vi "FPGA2_EPTDigChannels_eDIDS.vi"(0 "NI 9411-3/DI5:0":u8, 1 "VRHall-1.Data":T3 caption="VRHall_Data", 2 "9411-3.Invert":u8, 3 "VRHall-1.Invert":u8, 4 "9411-3.FilterValues":T2, 5 "VRHall-1.FilterValues":T4) -> (8 "9411-3.0.PPWData":T1, 9 "VRHall-1.1.PPWData":T1, 10 "9411-3.1.PPWData":T1, 11 "VRHall-1.2.PPWData":T1, 12 "9411-3.2.PPWData":T1, 13 "VRHall-1.3.PPWData":T1, 14 "9411-3.3.PPWData":T1, 15 "VRHall-1.4.PPWData":T1, 16 "9411-3.4.PPWData":T1, 17 "VRHall-1.5.PPWData":T1, 18 "9411-3.5.PPWData":T1, 19 "VRHall-1.6.PPWData":T1, 20 "9411-3.DigitalTriggers":bool[](array[boolean]), 21 "VRHall-1.DigitalTriggers":bool[](array[boolean]))   [LabVIEW 2015, in "ECS-FPGA.lvlib"]
uses:
  ECS-FPGA.lvlib
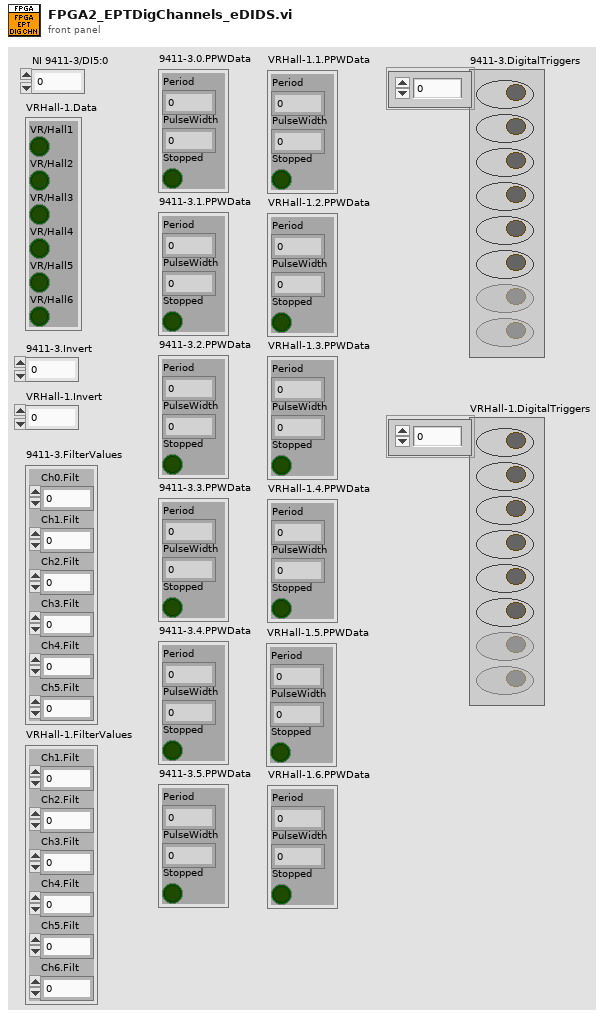
[diagram p1: front panel]
types:
  T1 = cluster{"Period":u32, "PulseWidth":u32, "Stopped":bool}
  T2 = cluster{"Ch0.Filt":u16, "Ch1.Filt":u16, "Ch2.Filt":u16, "Ch3.Filt":u16, "Ch4.Filt":u16, "Ch5.Filt":u16}
  T3 = cluster{"VR/Hall1":bool, "VR/Hall2":bool, "VR/Hall3":bool, "VR/Hall4":bool, "VR/Hall5":bool, "VR/Hall6":bool}
  T4 = cluster{"Ch1.Filt":u16, "Ch2.Filt":u16, "Ch3.Filt":u16, "Ch4.Filt":u16, "Ch5.Filt":u16, "Ch6.Filt":u16}
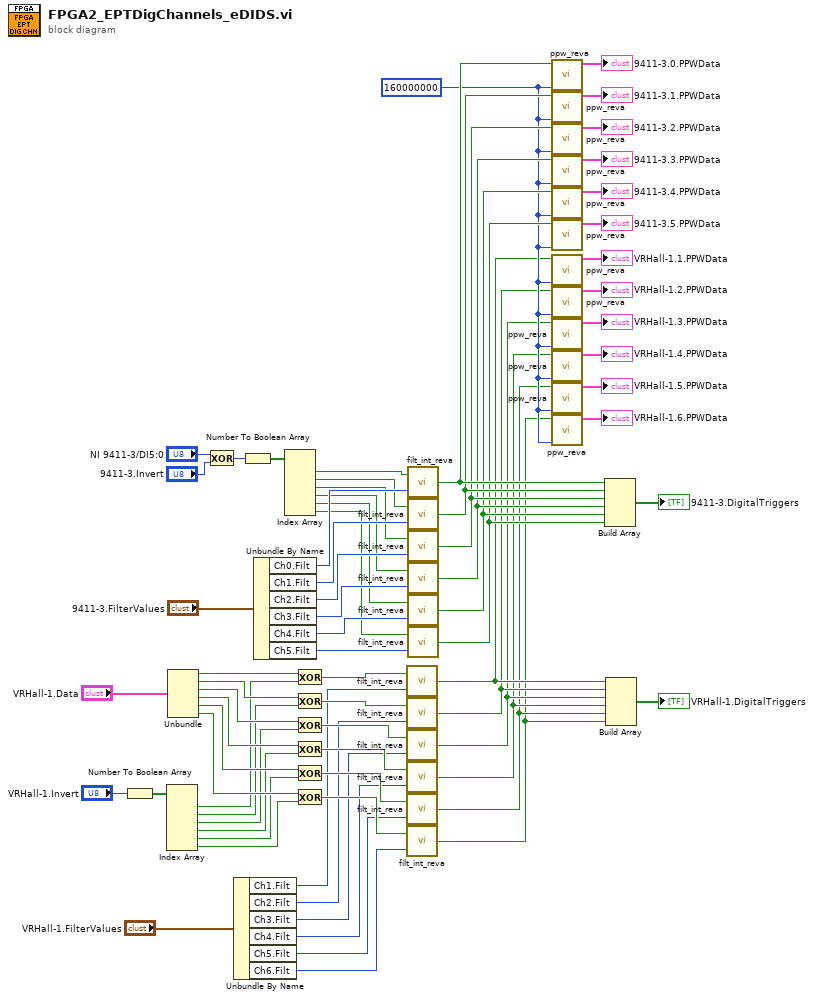
[diagram p0: block diagram]
diagram:
  w32 = u32 160000000 ("StopValue")
  n1 = Number To Boolean Array(number="VRHall-1.Invert") -> (Boolean array=w58:bool[])
  n2 = Index Array(array=w58) -> (element #1=w51:bool, element #2=w50:bool, element #3=w49:bool, element #4=w48:bool, element #5=w47:bool, element #6=w46:bool)  [unwired: 6 in]
  n3 = Unbundle("VRHall-1.Data") -> ("VR/Hall1"=w57:bool, "VR/Hall2"=w56:bool, "VR/Hall3"=w55:bool, "VR/Hall4"=w54:bool, "VR/Hall5"=w53:bool, "VR/Hall6"=w52:bool)
  n4 = Exclusive Or(1:"9411-3.Invert", 2:"NI 9411-3/DI5:0") -> (0:w41:u8)
  n5 = Unbundle By Name("VRHall-1.FilterValues") -> ("Ch1.Filt"=w25:u16, "Ch2.Filt"=w24:u16, "Ch3.Filt"=w23:u16, "Ch4.Filt"=w22:u16, "Ch5.Filt"=w21:u16, "Ch6.Filt"=w20:u16)
  n6 = Number To Boolean Array(number=w41) -> (Boolean array=w42:bool[])
  n7 = Unbundle By Name("9411-3.FilterValues") -> ("Ch0.Filt"=w65:u16, "Ch1.Filt"=w64:u16, "Ch2.Filt"=w63:u16, "Ch3.Filt"=w62:u16, "Ch4.Filt"=w61:u16, "Ch5.Filt"=w60:u16)
  n8 = Index Array(array=w42) -> (element #1=w40:bool, element #2=w39:bool, element #3=w38:bool, element #4=w37:bool, element #5=w36:bool, element #6=w35:bool)  [unwired: 6 in]
  n9 = Exclusive Or(1:w51, 2:w57) -> (0:w31:bool)
  n10 = Exclusive Or(1:w50, 2:w56) -> (0:w30:bool)
  n11 = Exclusive Or(1:w49, 2:w55) -> (0:w29:bool)
  n12 = Exclusive Or(1:w48, 2:w54) -> (0:w28:bool)
  n13 = Exclusive Or(1:w47, 2:w53) -> (0:w27:bool)
  n14 = Exclusive Or(1:w46, 2:w52) -> (0:w26:bool)
  n15 = call <vilib>:"filt_int_reva.vi"("FiltValue"=w25, "InpSig"=w31) -> ("OutSig"=w6:bool)
  n16 = call <vilib>:"filt_int_reva.vi"("FiltValue"=w24, "InpSig"=w30) -> ("OutSig"=w5:bool)
  n17 = call <vilib>:"filt_int_reva.vi"("FiltValue"=w23, "InpSig"=w29) -> ("OutSig"=w4:bool)
  n18 = call <vilib>:"filt_int_reva.vi"("FiltValue"=w22, "InpSig"=w28) -> ("OutSig"=w3:bool)
  n19 = call <vilib>:"filt_int_reva.vi"("FiltValue"=w21, "InpSig"=w27) -> ("OutSig"=w2:bool)
  n20 = call <vilib>:"filt_int_reva.vi"("FiltValue"=w20, "InpSig"=w26) -> ("OutSig"=w1:bool)
  n21 = call <vilib>:"filt_int_reva.vi"("FiltValue"=w65, "InpSig"=w40) -> ("OutSig"=w72:bool)
  n22 = call <vilib>:"filt_int_reva.vi"("FiltValue"=w64, "InpSig"=w39) -> ("OutSig"=w70:bool)
  n23 = call <vilib>:"filt_int_reva.vi"("FiltValue"=w63, "InpSig"=w38) -> ("OutSig"=w69:bool)
  n24 = call <vilib>:"filt_int_reva.vi"("FiltValue"=w62, "InpSig"=w37) -> ("OutSig"=w68:bool)
  n25 = call <vilib>:"filt_int_reva.vi"("FiltValue"=w61, "InpSig"=w36) -> ("OutSig"=w67:bool)
  n26 = call <vilib>:"filt_int_reva.vi"("FiltValue"=w60, "InpSig"=w35) -> ("OutSig"=w66:bool)
  n27 = call <vilib>:"ppw_reva.vi"("StopValue"=w32, "InpSig"=w72) -> ("PPWData"=→"9411-3.0.PPWData":T1)  [unwired: 2 in, 3 out]
  n28 = call <vilib>:"ppw_reva.vi"("StopValue"=w32, "InpSig"=w70) -> ("PPWData"=→"9411-3.1.PPWData":T1)  [unwired: 2 in, 3 out]
  n29 = call <vilib>:"ppw_reva.vi"("StopValue"=w32, "InpSig"=w69) -> ("PPWData"=→"9411-3.2.PPWData":T1)  [unwired: 2 in, 3 out]
  n30 = call <vilib>:"ppw_reva.vi"("StopValue"=w32, "InpSig"=w68) -> ("PPWData"=→"9411-3.3.PPWData":T1)  [unwired: 2 in, 3 out]
  n31 = call <vilib>:"ppw_reva.vi"("StopValue"=w32, "InpSig"=w67) -> ("PPWData"=→"9411-3.4.PPWData":T1)  [unwired: 2 in, 3 out]
  n32 = call <vilib>:"ppw_reva.vi"("StopValue"=w32, "InpSig"=w66) -> ("PPWData"=→"9411-3.5.PPWData":T1)  [unwired: 2 in, 3 out]
  n33 = call <vilib>:"ppw_reva.vi"("StopValue"=w32, "InpSig"=w6) -> ("PPWData"=→"VRHall-1.1.PPWData":T1)  [unwired: 2 in, 3 out]
  n34 = call <vilib>:"ppw_reva.vi"("StopValue"=w32, "InpSig"=w5) -> ("PPWData"=→"VRHall-1.2.PPWData":T1)  [unwired: 2 in, 3 out]
  n35 = call <vilib>:"ppw_reva.vi"("StopValue"=w32, "InpSig"=w4) -> ("PPWData"=→"VRHall-1.3.PPWData":T1)  [unwired: 2 in, 3 out]
  n36 = call <vilib>:"ppw_reva.vi"("StopValue"=w32, "InpSig"=w3) -> ("PPWData"=→"VRHall-1.4.PPWData":T1)  [unwired: 2 in, 3 out]
  n37 = call <vilib>:"ppw_reva.vi"("StopValue"=w32, "InpSig"=w2) -> ("PPWData"=→"VRHall-1.5.PPWData":T1)  [unwired: 2 in, 3 out]
  n38 = call <vilib>:"ppw_reva.vi"("StopValue"=w32, "InpSig"=w1) -> ("PPWData"=→"VRHall-1.6.PPWData":T1)  [unwired: 2 in, 3 out]
  n39 = Build Array(w72, w70, w69, w68, w67, w66) -> (→"9411-3.DigitalTriggers":bool[])
  n40 = Build Array(w6, w5, w4, w3, w2, w1) -> (→"VRHall-1.DigitalTriggers":bool[])
